vi "3D-DateCollect.vi"(11 "Start Time":string) -> (3 "Date Message":string[](array[string]))   [LabVIEW 2015]
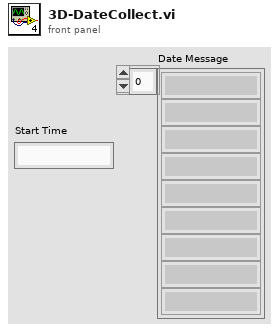
[diagram p1: front panel]
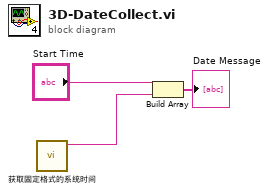
[diagram p0: block diagram]
diagram:
  n1 = call "获取固定格式的系统时间.vi"() -> ("日期/时间字符串"=w2:string)  [unwired: 10 in, 1 out]
  n2 = Build Array("Start Time", w2) -> (→"Date Message":string[])
